vi "執行測試.vi"() -> ()   [LabVIEW 2019]
uses:
  <vilib>/Instr/_visa.llb/VISA Configure Serial Port (Instr).vi
panel:
  out "?":string
  out "String":string
  in  "stop":bool
  in  "LF":bool
  in  "LO":bool
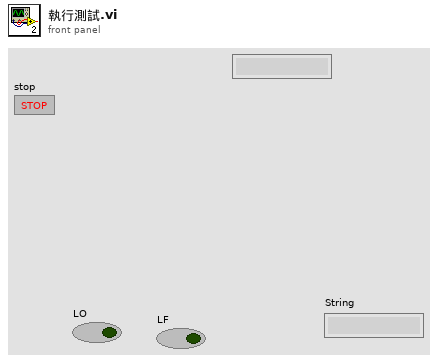
[diagram p1: front panel]
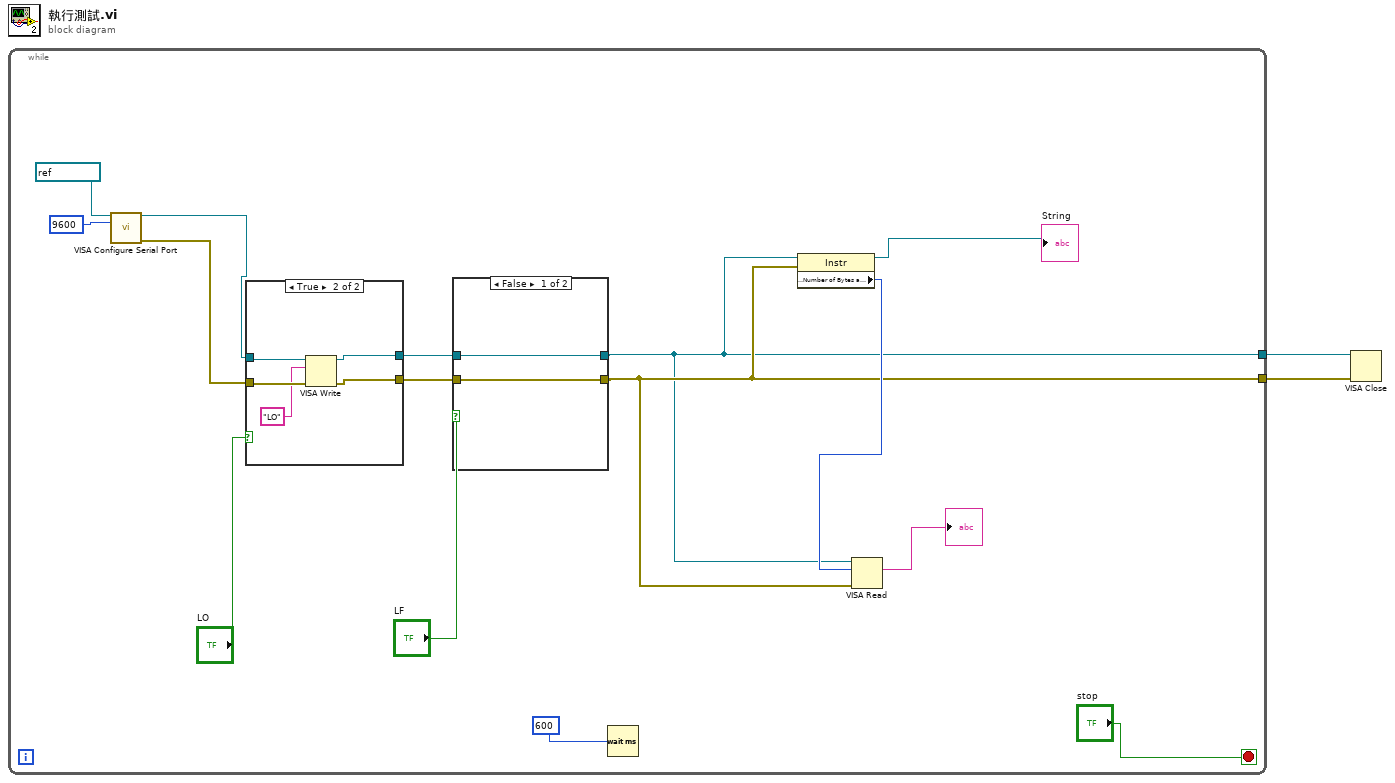
[diagram p0: block diagram]
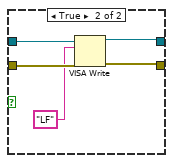
[diagram p2: hidden frame]
diagram:
  n1 = while {
    tunnel: [w7] -> w2
    tunnel: [w8] -> w1
    stop <- "stop" stop-if-true
    n2 = call-poly "VISA Configure Serial Port"("VISA resource name"=refnum<visa-resource-name> "COM6", "baud rate (9600)"=u32 9600) -> ("VISA resource name out"=w6:refnum<visa-resource-name>, "error out"=w5:errorcluster)  [unwired: 12 in]
    n3 = case shown="True" "LO" {
      tunnel: w6 -> [w26 w31]
      tunnel: w5 -> [w25 w28]
      tunnel: [w26 w30] -> w17
      tunnel: [w25 w29] -> w16
      frame False {
      }
      frame True {
        n4 = VISA Write(VISA resource name=w31, write buffer="LO", error in (no error)=w28) -> (VISA resource name out=w30:refnum<visa-resource-name>, error out=w29:errorcluster)  [unwired: 1 out]
      }
    }
    n5 = case shown="False" "LF" {
      tunnel: w17 -> [w19 w24]
      tunnel: w16 -> [w18 w22]
      tunnel: [w19 w23] -> w7
      tunnel: [w18 w21] -> w8
      frame False {
      }
      frame True {
        n6 = VISA Write(VISA resource name=w24, write buffer="LF", error in (no error)=w22) -> (VISA resource name out=w23:refnum<visa-resource-name>, error out=w21:errorcluster)  [unwired: 1 out]
      }
    }
    n7 = Wait (ms)(milliseconds to wait=u32 600) -> ()  [unwired: 1 out]
    n8 = property class="Instr"(reference=w7, error in=w8) -> (reference out=→"String":refnum<visa-resource-name>, "Serial Settings:Number of Bytes at Serial Port"=w10:u32)  [unwired: 1 out]
    n9 = VISA Read(VISA resource name=w7, byte count=w10, error in (no error)=w8) -> (read buffer=→"?":string)  [unwired: 3 out]
  }
  n10 = VISA Close(VISA resource name=w2, error in (no error)=w1) -> ()  [unwired: 1 out]
